vi "Result.Attribute Look Up Limits.vi"(0 "Attribute":T1 {"Status" items=["LOG", "PASS", "FAIL", "ERROR"]}, 4 "Limits":variant) -> (5 "Measurement Out":T1 {"Status" items=["LOG", "PASS", "FAIL", "ERROR"]})   [LabVIEW 2018]
uses:
  Result.Attribute.ctl
  Result.Measurement and Attribute Item Status.ctl
  Result.Test Limit Item.ctl
  Result.Limit Type.ctl
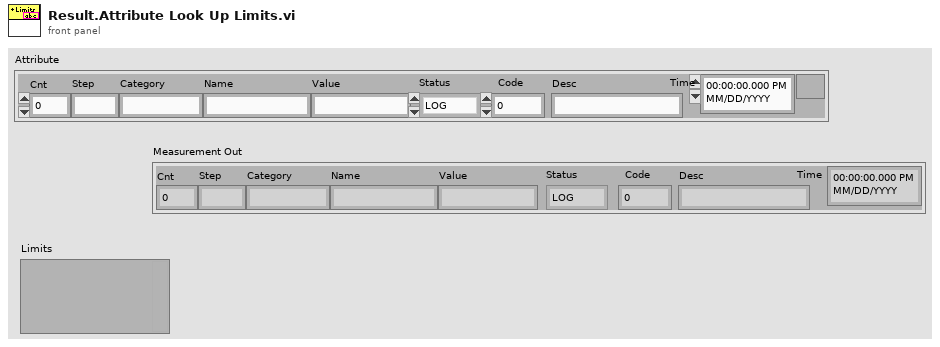
[diagram p1: front panel]
types:
  T1 = typedef "Result.Attribute.ctl" = cluster{"Cnt":i32, "Step":string, "Category":string, "Name":string, "Value":string, "Status":T2, "Code":i32, "Desc":string, "Time":timestamp}
  T2 = typedef "Result.Measurement and Attribute Item Status.ctl" = i32
  T3 = typedef "Result.Test Limit Item.ctl" = cluster{"Name":string, "LimType":T4, "LL":string, "UL":string, "Units":string, "FailCode":i32, "FailDesc":string}
  T4 = typedef "Result.Limit Type.ctl" = enum16{"None", "EQ", "NE", "GT", "LT", "GE", "LE", "GTLT", "GELE", "GELT", "GTLE", "LTGT", "LEGE", "LEGT", "LTGE"}
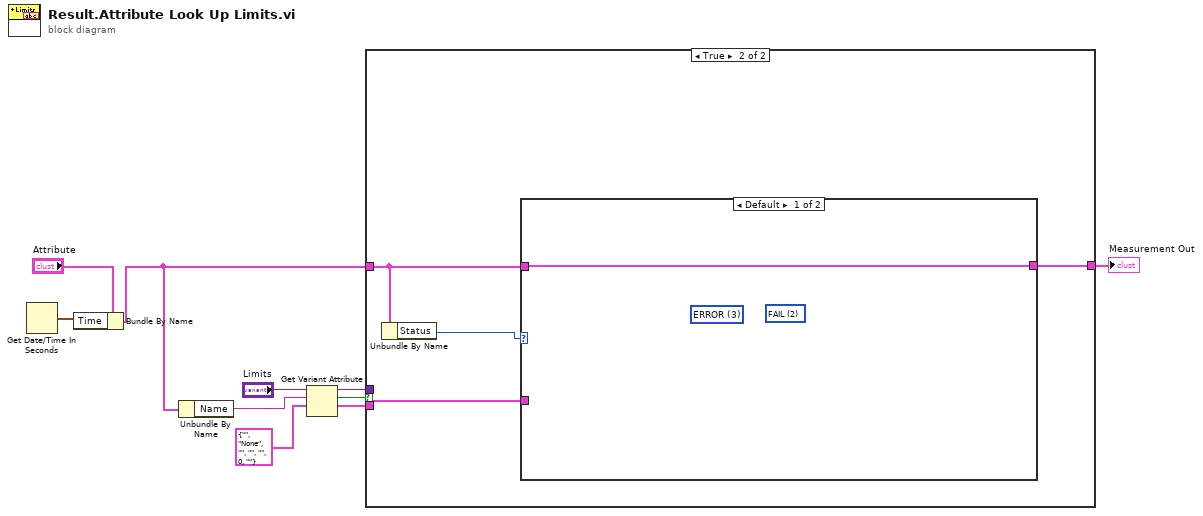
[diagram p0: block diagram]
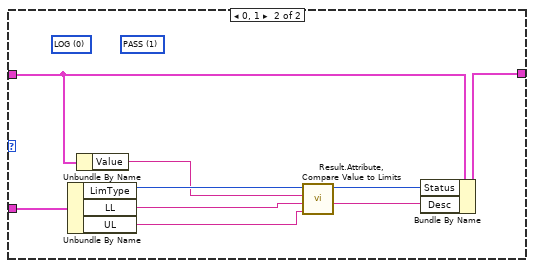
[diagram p3: hidden frame]
diagram:
  n1 = Get Date/Time In Seconds() -> (seconds since 1Jan1904=w3:timestamp)
  n2 = Bundle By Name(cluster="Attribute", "Time"=w3) -> (w1:T1)
  n3 = Unbundle By Name(w1) -> ("Name"=w9:string)
  n4 = Get Variant Attribute(Variant="Limits", name=w9, default value (empty Variant)=T3 {"Name"="", "LimType"=enum."None", "LL"="", "UL"="", "Units"="", "FailCode"=0, "FailDesc"=""} ("Result.Test Limit Item")) -> (duplicate Variant=w6:variant, found=w7:bool, value=w5:T3)  [unwired: 1 in, 1 out]
  n5 = case shown="True" w7 {
    tunnel: w6 -> [_ _]
    tunnel: w5 -> [_ w15]
    tunnel: w1 -> [w11 w13]
    tunnel: [w11 w14] -> w4
    frame False {
      # "If not found use None"
    }
    frame True {
      n6 = Unbundle By Name(w13) -> ("Status"=w12:T2)
      n7 = case shown="Default" w12 {
        tunnel: w15 -> [_ w25]
        tunnel: [w16 w23] -> w14
        tunnel: w13 -> [w16 w17]
        frame Default {
          (unwired) T2 2 items=["LOG", "PASS", "FAIL", "ERROR"] ("y")
          (unwired) T2 3 items=["LOG", "PASS", "FAIL", "ERROR"] ("y")
        }
        frame 0, 1 {
          (unwired) T2 1 items=["LOG", "PASS", "FAIL", "ERROR"] ("y")
          (unwired) T2 0 items=["LOG", "PASS", "FAIL", "ERROR"] ("y")
          n8 = Unbundle By Name(w25) -> ("LimType"=w22:T4, "LL"=w20:string, "UL"=w19:string)
          n9 = Unbundle By Name(w17) -> ("Value"=w21:string)
          n10 = call "Result.Attribute, Compare Value to Limits.vi"("UL"=w19, "LL"=w20, "Value"=w21, "LimType"=w22) -> ("Desc"=w18:string, "Status"=w24:T2)  [unwired: 6 in]
          n11 = Bundle By Name(cluster=w17, "Status"=w24, "Desc"=w18) -> (w23:T1)
        }
      }
    }
  }
  "Measurement Out" <- w4
